vi "Initialize.vi"(8 "error in (no error)":errorcluster, 10 "Subpnl":refnum<vi>, 11 "ViewMgr in":refnum<class "ViewMgr.lvclass">) -> (0 "error out":errorcluster, 3 "ViewMgr out":refnum<class "ViewMgr.lvclass">)   [LabVIEW 2020, in "CSM-TagDBDisplayContainer.lvlib" / "ViewMgr.lvclass"]
uses:
  ViewMgr.lvclass
  ViewMgr.lvclass/ViewMgr.ctl
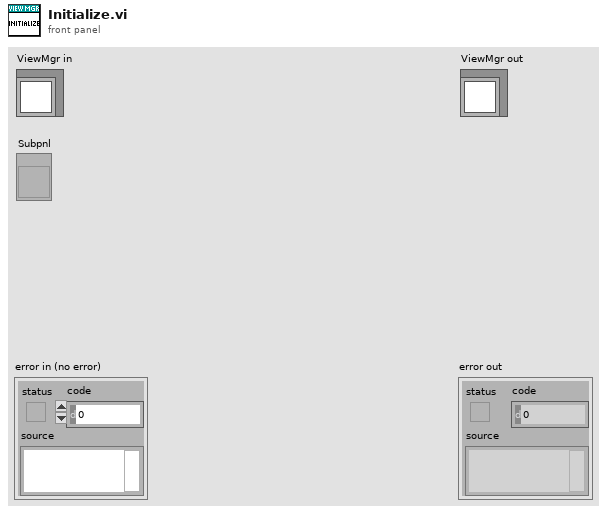
[diagram p1: front panel]
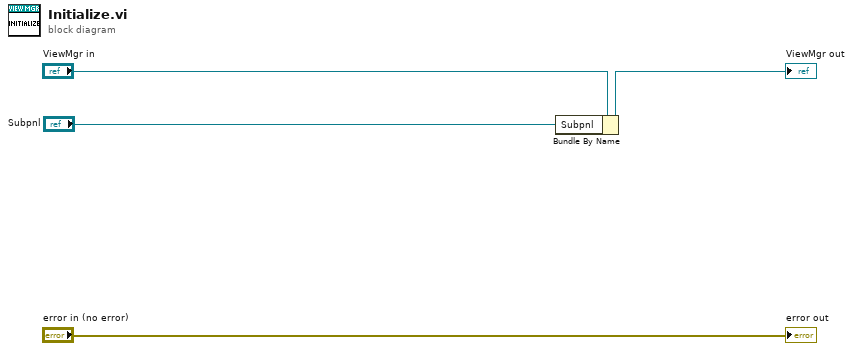
[diagram p0: block diagram]
diagram:
  n1 = Bundle By Name(cluster="ViewMgr in", "Subpnl"="Subpnl") -> (→"ViewMgr out":refnum<class "ViewMgr.lvclass">)
  "error out" <- "error in (no error)"
